vi "_Create Resp Queue.vi"(7 "max queue size (-1, unlimited)":i32=-1, 8 "error in (no error)":errorcluster, 9 "create if not found? (T)":bool=TRUE) -> (0 "error out":errorcluster, 1 "created new?":bool, 3 "queue out":refnum<queue>)   [LabVIEW 2014, in "JKI State Machine++.lvlib"]
uses:
  JKI State Machine++.lvlib
  Typedef/_Cross JKISM State Response.ctl
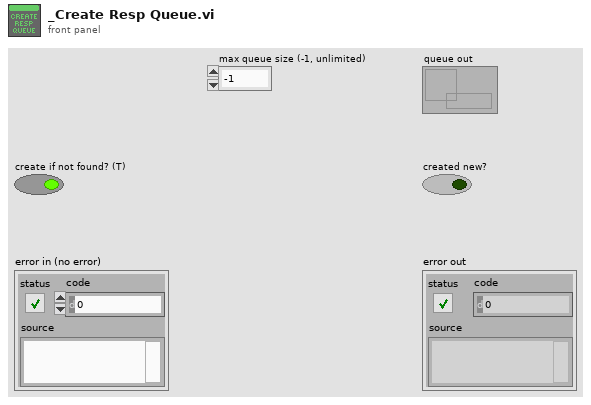
[diagram p1: front panel]
types:
  T1 = typedef "JKI State Machine++.lvlib/_Cross JKISM State Response.ctl" = cluster{"error":errorcluster, "Response Data":string, "From Who":string}
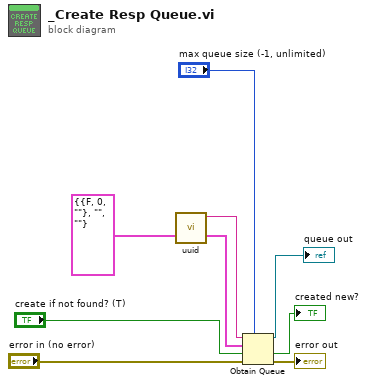
[diagram p0: block diagram]
diagram:
  n1 = call "uuid.vi"() -> ("UUID"=w1:string)  [unwired: 11 in]
  n2 = Obtain Queue(max queue size (-1, unlimited)="max queue size (-1, unlimited)", name (unnamed)=w1, element data type=T1 {"error"={"status"=FALSE, "code"=0, "source"=""}, "Response Data"="", "From Who"=""} ("Cross JKI State Machine Response"), create if not found? (T)="create if not found? (T)", error in (no error)="error in (no error)") -> (queue out=→"queue out":refnum<queue>, created new?=→"created new?":bool, error out=→"error out":errorcluster)
